vi "Linelización.vi"(8 "Longitud":i32, 9 "Indice":i32, 10 "Array Y":dbl[](array[numeric]), 11 "Array X":dbl[](array[numeric])) -> (1 "intercept":dbl, 2 "slope":dbl, 3 "Array out":dbl[](array[numeric]))   [LabVIEW 2017]
uses:
  <vilib>/Analysis/NI_AALPro.lvlib
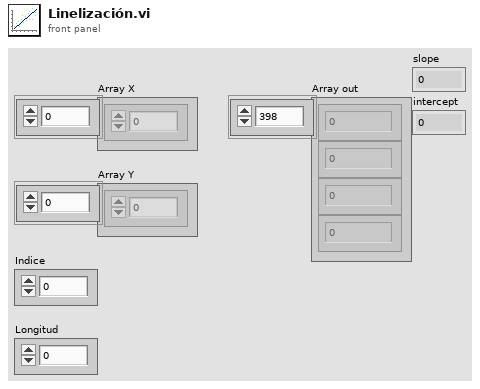
[diagram p1: front panel]
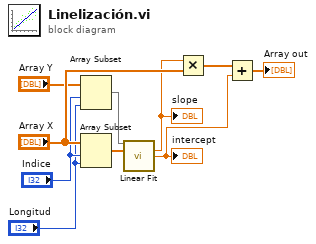
[diagram p0: block diagram]
diagram:
  n1 = Array Subset(array="Array Y", index="Indice", length="Longitud") -> (w5:dbl[])
  n2 = Array Subset(array="Array X", index="Indice", length="Longitud") -> (w3:dbl[])
  n3 = call <vilib>:"Linear Fit.vi"("Y"=w5, "X"=w3) -> ("slope"=w6:dbl, "intercept"=w9:dbl)  [unwired: 9 in, 3 out]
  "slope" <- w6
  "intercept" <- w9
  n4 = Multiply(x=w6, y="Array X") -> (x*y=w8:dbl[])
  n5 = Add(x=w8, y=w9) -> (x+y=→"Array out":dbl[])
